vi "analog- input1.vi"() -> ()   [LabVIEW 2016]
doc: "이 예제는 컴퓨터 메모리의 버퍼로부터 정해진 수의 데이터를 생성하는 방법을 보여줍니다."
uses:
  <vilib>/Utility/error.llb/DialogType.ctl
  <vilib>/DAQmx/read.llb/DAQmx Read (Analog DBL 1Chan 1Samp).vi
  <vilib>/DAQmx/create/channels.llb/DAQmx Create Channel (AI-Voltage-Basic).vi
  <vilib>/DAQmx/miscellaneous.llb/DAQmx Fill In Error Info.vi
panel:
  out "웨이브폼 차트":dbl(graph)
  in  "input terminal configuration":i32(ring)=-1 items=["기본"=-1, "RSE"=10083, "NRSE"=10078, "차동"=10106, "유사 차동"=12529]
  out "data":dbl caption="dateta" format="%0.2f"
  in  "최대 전압":dbl=5.0
  in  "최소 전압":dbl=-5.0
  in  "물리적 채널":tag="Dev1/ao0"
  # "channel"
  # "input terminal configuration"
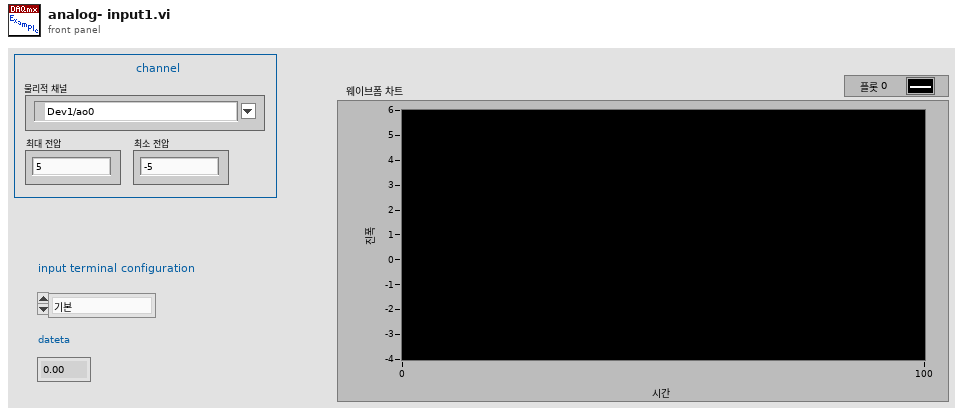
[diagram p1: front panel]
types:
  T1 = typedef "DialogType.ctl" = u16
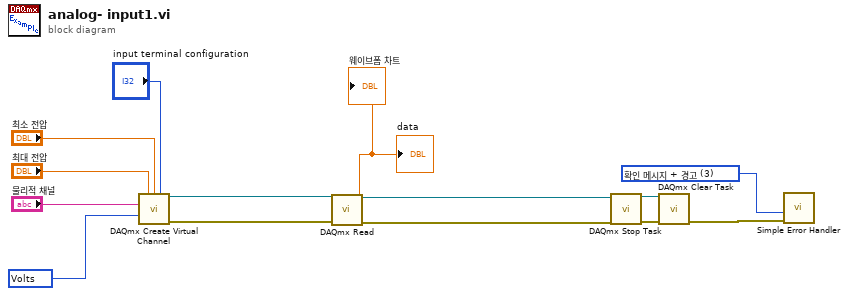
[diagram p0: block diagram]
diagram:
  w4 = 10348 items=["Volts"=10348, "사용자 스케일로부터"=10065] ("units")
  w8 = T1 3 items=["대화 상자 없음", "확인 메시지", "메시지 지속 또는 정지", "확인 메시지 + 경고", "지속/정지 + 경고"] ("대화 상자 타입 (확인 메시지:1)")
  n1 = call-poly <vilib>:"DAQmx Create Virtual Channel.vi"("maximum value"="최대 전압", "minimum value"="최소 전압", "input terminal configuration"="input terminal configuration", "physical channels"="물리적 채널", "units"=w4) -> ("task out"=w5:refnum<k21>, "error out"=w7:errorcluster)  [unwired: 9 in]
  n2 = call-poly <vilib>:"DAQmx Read.vi"("task/channels in"=w5, "error in"=w7) -> ("task out"=w2:refnum<k21>, "data"=→"data" →"웨이브폼 차트":dbl, "error out"=w6:errorcluster)  [unwired: 11 in]
  n3 = call <vilib>:"DAQmx Stop Task.vi"("task/channels in"=w2, "error in"=w6) -> ("task out"=w10:refnum<k21>, "error out"=w9:errorcluster)  [unwired: 12 in]
  n4 = call <vilib>:"DAQmx Clear Task.vi"("task in"=w10, "error in"=w9) -> ("error out"=w14:errorcluster)  [unwired: 13 in]
  n5 = call <vilib>:"Simple Error Handler.vi"("type of dialog (OK msg:1)"=w8, "error in (no error)"=w14) -> ()  [unwired: 3 in, 5 out]
